vi "Enqueue.vi"(8 "error in (no error)":errorcluster, 10 "Message":refnum<class "Message.lvclass">, 11 "Transporter in":refnum<class "Transporter.lvclass">) -> (0 "error out":errorcluster, 3 "Transporter out":refnum<class "Transporter.lvclass">)   [LabVIEW 2021, in "Msn Trasnsportation Library 1.lvlib" / "Transporter.lvclass"]
uses:
  Transporter.lvclass
  Message.lvclass
  Transporter.lvclass/Transporter.ctl
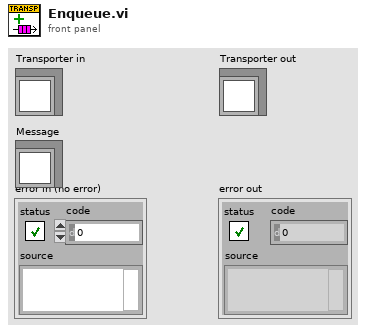
[diagram p1: front panel]
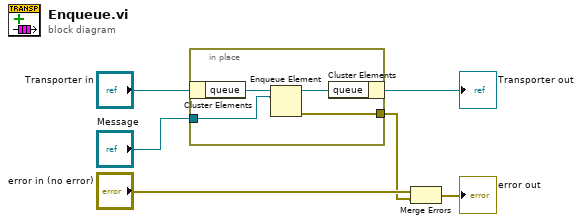
[diagram p0: block diagram]
diagram:
  n1 = in-place {
    in-place-border: [w7] -> w2
    in-place-border: "Message" -> [w6]
    n2 = in-place-cluster #1("Transporter in") -> ("queue"=w9:refnum<queue>)
    n3 = Enqueue Element(queue=w9, element=w6) -> (queue out=w8:refnum<queue>, error out=w7:errorcluster)  [unwired: 2 in, 1 out]
    n4 = in-place-cluster #1("queue"=w8) -> ()  [unwired: 1 out]
  }
  n5 = Merge Errors("error in (no error)", w2) -> (→"error out":errorcluster)
  "Transporter out" <- "Transporter in"
